vi "Two Color Servo Camera.vi"() -> ()   [LabVIEW 2013]
doc: "<B>Two Color Servo Camera </B> tracks a pink/green object by moving a gimbal mounted camera to keep the object centered in the image. It assumes the camera is mounted upright, and that the DS is connected. It is written to control two servos, but will work fine with one."
uses:
  <vilib>/addons/control/pid/pid.llb/PID Control Input Filter (DBL).vi
  <vilib>/Rock Robotics/WPI/Camera/WPI_CameraImageSize.ctl
  <vilib>/Rock Robotics/WPI/Camera/WPI_CameraWhite Balance Values.ctl
  <vilib>/Rock Robotics/WPI/Camera/WPI_CameraExposure Values.ctl
  Control Statesv1.ctl
  <vilib>/Rock Robotics/SystemInterfaces/DIO/FPGA_DIOPWMChannel.ctl
  <vilib>/Rock Robotics/WPI/Camera/WPI_CameraFrameRate.ctl
panel:
  in  "stop":bool
  in  "Frame Rate (fps)":T1=15 min=1 max=30
  out "Target":T2
  in  "Brightness":i32=40 min=0 max=100
  out "fps":dbl
  in  "Pink First":bool=TRUE
  in  "Friend Colors":enum32{"Pink over Green", "Green over Pink"}(radio)
  in  "Adv Processing Inputs":T3={"SubRect"={"Left"=0, "Top"=0, "Right"=640, "Bottom"=480}, "Decimate"={"H"=1, "V"=1}} {"Decimate"."V" min=1 max=1000; "Decimate"."H" min=1 max=1000}
  in  "Color Thresholds":T4(array[cluster])=[{"Hue"={"Min"=220, "Max"=255}, "Sat"={"Min"=75, "Max"=255}, "Luma"={"Min"=85, "Max"=255}}, {"Hue"={"Min"=55, "Max"=125}, "Sat"={"Min"=58, "Max"=255}, "Luma"={"Min"=92, "Max"=255}}]
  in  "Image Processing Limits":T5={"Find Foe"=TRUE, "Max Time (sec)"=0.25, "Min Obj Size %"=0.005, "Max Particles"=10}
  in  "Operation":enum32{"Camera Display", "Gimbal Track"}(radio)
  out "Servo Tracking State":T7
  in  "Servo Positions":cluster{"X":dbl, "Y":dbl}={"X"=85.52840986947938, "Y"=85.0} {"Y" scale=0.0..170.0; "X" scale=0.0..170.0}
  in  "Y Channel":T8=enum."PWM 10"
  in  "Servo Sleep (ms)":u32=20
  in  "X Channel":T8=enum."PWM 9"
  in  "Smooth":bool=TRUE
  out "Mask":T9(plugin-control)
  in  "Display Mask":bool=TRUE
  out "Camera Image":T9(plugin-control)
  # "This example will track a pink/green object by moving a gimbal mounted camera to keep the object centered in the image. It assumes the camera is mounted upright, and that the DS is connected. It is written to control two servos, but will work fine with one.\n\nThe setup code for the camera assumes that it is plugged into the switch and set to 10.te.am.11. To use on port 2 of an 8-slot controller, change the IP address wired into open.\n\nTo fine tune the colors, you may find it easiest to set the Operation control to Camera Display. This way the servos will not update and you can experiment with the colors or camera brightness  to get a good mask. Once the color thresholds are set appropriately for the object you are tracking, switch Operation to Gimbal Track."
  # "Servo Settings"
  # "Limit processing to a friend or foe,\nto a maximum amount of time,\nto particles above a minimum\nsize, and to a maximum number of color\nparticles"
  # "SubRect and decimate are used\nto limit the number of pixels to\nprocess. SubRect will for example\nextract the upper half of the\nimage. Decimate shrinks the image\nby for example leaving out every\nother row if V is set to 2."
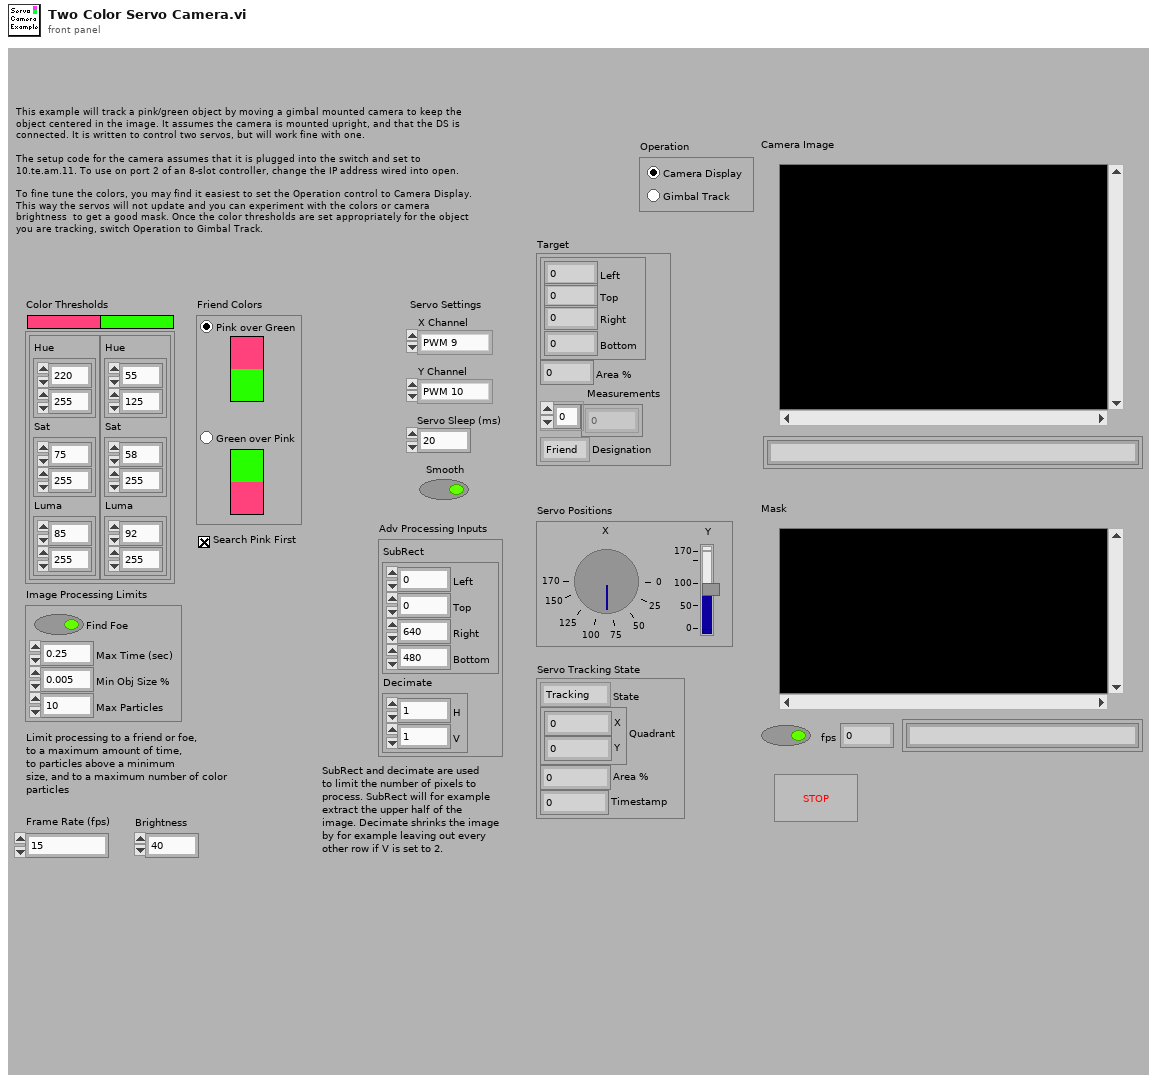
[diagram p1: front panel]
types:
  T1 = typedef "WPI_CameraFrameRate.ctl" = u32
  T2 = cluster{"Rectangle":cluster{"Left":i32, "Top":i32, "Right":i32, "Bottom":i32}, "Area %":dbl, "Measurements":dbl[], "Designation":enum16{"Friend", "Foe"}}
  T3 = cluster{"SubRect":cluster{"Left":i32, "Top":i32, "Right":i32, "Bottom":i32}, "Decimate":cluster{"H":i32, "V":i32}}
  T4 = cluster{"Hue":cluster{"Min":i32, "Max":i32}, "Sat":cluster{"Min":i32, "Max":i32}, "Luma":cluster{"Min":i32, "Max":i32}}[]
  T5 = cluster{"Find Foe":bool, "Max Time (sec)":dbl, "Min Obj Size %":sgl, "Max Particles":i32}
  T6 = typedef "Control Statesv1.ctl" = enum16{"Tracking", "Lost Small", "Lost-Patience", "Search-Begin", "Searching", "Lost - Edge"}
  T7 = cluster{"State":T6, "Quadrant":cluster{"X":i32, "Y":i32}, "Area %":dbl, "Timestamp":u32}
  T8 = typedef "FPGA_DIOPWMChannel.ctl" = enum8{"PWM 1", "PWM 2", "PWM 3", "PWM 4", "PWM 5", "PWM 6", "PWM 7", "PWM 8", "PWM 9", "PWM 10", "Invalid"}
  T9 = typedef "IMAQ Image.ctl" = refnum<image>
  T10 = typedef "WPI_CameraExposure Values.ctl" = enum16{"Auto", "Flicker-free 50 Hz", "Flicker-free 60 Hz", "Hold current"}
  T11 = typedef "WPI_CameraWhite Balance Values.ctl" = enum16{"Auto", "Fixed indoor", "Fixed outdoor 1", "Fixed outdoor 2", "Fixed fluorescent 1", "Fixed fluorescent 2", "Hold current"}
  T12 = typedef "WPI_CameraImageSize.ctl" = enum16{"640x480", "320x240", "160x120"}
  T13 = typedef "WPI_CameraDevRef.ctl" = cluster{"Camera Address":string, "CameraStatus":errorcluster, "Acquire Image Notifier":refnum<notifier>}
  T14 = cluster{"Image Processing Limits":cluster{"Find Foe":bool, "Max Time (sec)":dbl, "Min Obj Size %":sgl, "Max Particles":i32}, "Image Size":T12, "Pink First":bool}
  T15 = cluster{"State":T6, "Quadrant":cluster{"X":i32, "Y":i32}, "Area":dbl, "millisecond timer value":u32}
  T16 = typedef "WPI_ServoDeviceRef.ctl" = cluster{"DeviceStatus":errorcluster, "Digital Module":T17, "PWM Channel":T8, "DeadBand":T18}
  T17 = typedef "FPGA_TypedefDigitalModule.ctl" = enum16{"Digital Module 1", "Digital Module 2"}
  T18 = typedef "WPI_PWMDeadband.ctl" = cluster{"Name":string, "maxPositivePwm":i32, "minPositivePwm":i32, "centerPwm":i32, "maxNegativePwm":i32, "minNegativePwm":i32, "angularRange":u16}
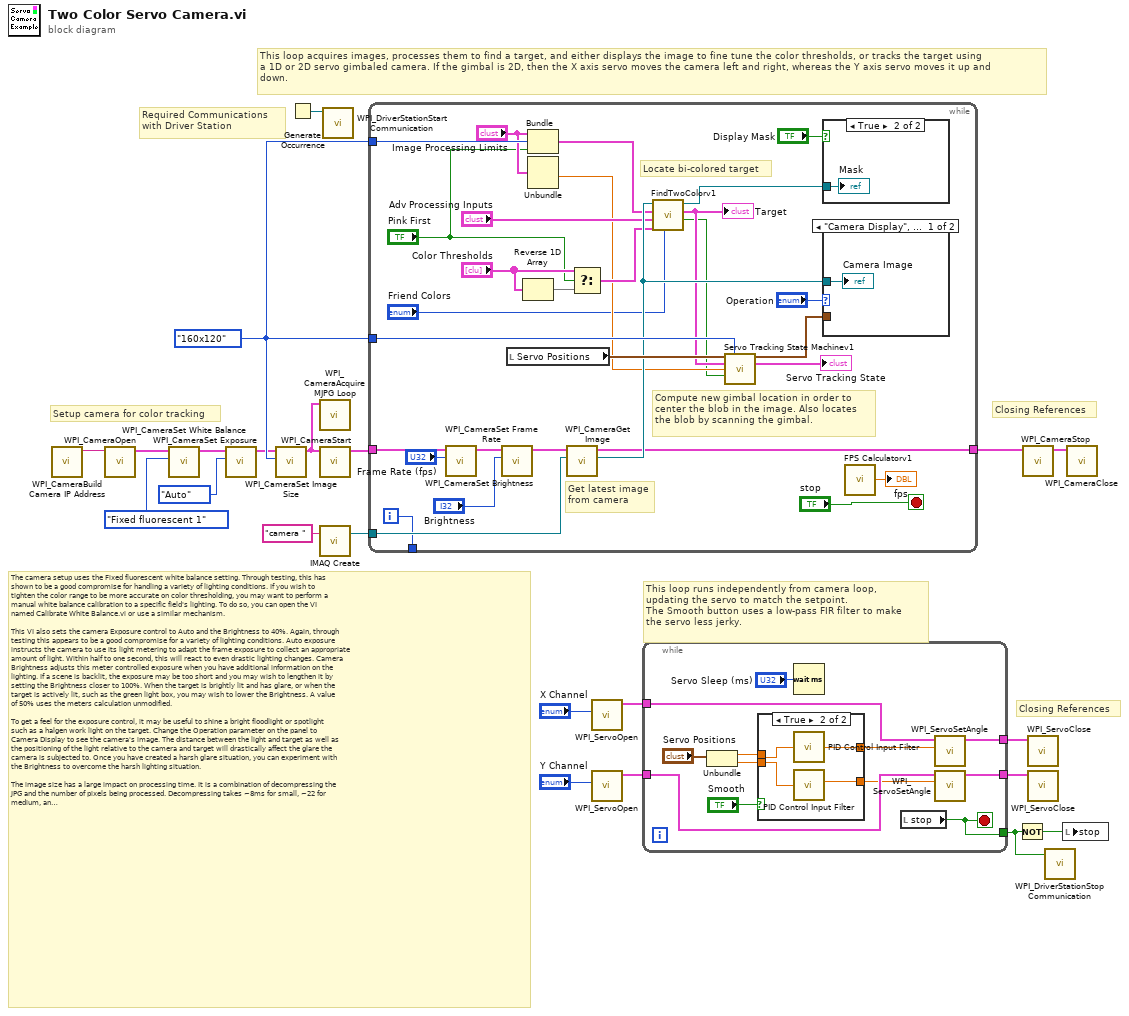
[diagram p0: block diagram]
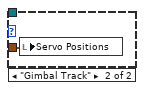
[diagram p3: hidden frame]
diagram:
  w13 = WPI_CameraImageSize."160x120" ("Image Size")
  # "Closing References"
  # "The camera setup uses the Fixed fluorescent white balance setting. Through testing, this has\nshown to be a good compromise for handling a variety of lighting conditions. If you wish to\ntighten the color range to be more accurate on color thresholding, you may want to perform a\nmanual white balance calibration to a specific field's lighting. To do so, you can open the VI\nnamed Calibrate White Balance.vi or use a similar mechanism.\n\nThis VI also sets the camera Exposure control to Auto and the Brightness to 40%. Again, through\ntesting this appears to be a good compromise for a variety of lighting conditions. Auto exposure\ninstructs the camera to use its light metering to adapt the frame exposure to collect an appropriate\namount of light. Within half to one second, this will react to even drastic lighting changes. Camera\nBrightness adjusts this meter controlled exposure when you have additional information on the\nlighting. If a scene is backlit, the exposure may be too short and you may wish to lengthen it by\nsetting the Brightness closer to 100%. When the target is brightly lit and has glare, or when the\ntarget is actively lit, such as the green light box, you may wish to lower the Brightness. A value\nof 50% uses the meters calculation unmodified.\n\nTo get a feel for the exposure control, it may be useful to shine a bright floodlight or spotlight\nsuch as a halgen work light on the target. Change the Operation parameter on the panel to\nCamera Display to see the camera's image. The distance between the light and target as well as\nthe positioning of the light relative to the camera and target will drastically affect the glare the\ncamera is subjected to. Once you have created a harsh glare situation, you can experiment with\nthe Brightness to overcome the harsh lighting situation.\n\nThe image size has a large impact on processing time. It is a combination of decompressing the\nJPG and the number of pixels being processed. Decompressing takes ~8ms for small, ~22 for\nmedium, and ~100 for large. After decompression, the processing time for locating targets is\nlargely related to the number of pixels. You may want to use the subRect or decimation factors\nto control the pixels being processed. Lower resolution or decimated images will be less effective\nat finding targets at distance."
  # "Closing References"
  # "This loop acquires images, processes them to find a target, and either displays the image to fine tune the color thresholds, or tracks the target using\na 1D or 2D servo gimbaled camera. If the gimbal is 2D, then the X axis servo moves the camera left and right, whereas the Y axis servo moves it up and\ndown."
  # "This loop runs independently from camera loop,\nupdating the servo to match the setpoint.\nThe Smooth button uses a low-pass FIR filter to make\nthe servo less jerky."
  # "Setup camera for color tracking"
  # "Required Communications\nwith Driver Station"
  n1 = call <vilib>:"WPI_CameraBuild Camera IP Address.vi"() -> ("Camera Address"=w3:string)  [unwired: 11 in]
  n2 = call <vilib>:"WPI_CameraOpen.vi"("Camera Address"=w3) -> ("CameraDevRef"=w11:T13)  [unwired: 1 in, 9 out]
  n3 = call <vilib>:"WPI_CameraSet White Balance.vi"("White Balance"=WPI_CameraWhite_Balance_Values."Fixed fluorescent 1", "CameraDevRef"=w11) -> ("CameraDevRef Out"=w9:T13)  [unwired: 1 in, 8 out]
  n4 = call <vilib>:"WPI_CameraSet Exposure.vi"("Exposure"=WPI_CameraExposure_Values."Auto", "CameraDevRef"=w9) -> ("CameraDevRef Out"=w4:T13)  [unwired: 1 in, 8 out]
  n5 = call <vilib>:"WPI_CameraSet Image Size.vi"("Image Size"=w13, "CameraDevRef"=w4) -> ("CameraDevRef Out"=w5:T13)  [unwired: 1 in, 8 out]
  n6 = Generate Occurrence() -> (w12:refnum<k4>)
  n7 = call <vilib>:"WPI_CameraAcquire MJPG Loop.vi"("CameraDevRef"=w5) -> ()  [unwired: 11 in]
  n8 = call <vilib>:"WPI_CameraStart.vi"("CameraDevRef"=w5) -> ("CameraDevRef Out"=w15:T13)  [unwired: 1 in, 9 out]
  n9 = call "IMAQ Create"("Image Name"="camera ") -> ("New Image"=w16:T9)  [unwired: 3 in, 2 out]
  n10 = call <vilib>:"WPI_DriverStationStart Communication.vi"("occurrence"=w12) -> ()  [unwired: 11 out]
  n11 = while {
    tunnel: w15 -> [w27]
    tunnel: [w36] -> w14
    tunnel: w16 -> [w52]
    tunnel: w13 -> [w48]
    tunnel: w13 -> [w39]
    tunnel: [w24] -> _
    i -> [w24]
    stop <- "stop" stop-if-true
    # "Locate bi-colored target"
    # "Compute new gimbal location in order to\ncenter the blob in the image. Also locates\nthe blob by scanning the gimbal."
    # "Get latest image\nfrom camera"
    n12 = call <vilib>:"WPI_CameraSet Frame Rate.vi"("Frame Rate (fps)"="Frame Rate (fps)", "CameraDevRef"=w27) -> ("CameraDevRef Out"=w26:T13)  [unwired: 1 in, 8 out]
    n13 = call <vilib>:"WPI_CameraSet Brightness.vi"("Brightness"="Brightness", "CameraDevRef"=w26) -> ("CameraDevRef Out"=w33:T13)  [unwired: 1 in, 8 out]
    n14 = local read "Servo Positions"() -> (w49:cluster{"X":dbl, "Y":dbl})
    n15 = Reverse 1D Array(array="Color Thresholds") -> (reversed array=w41:T4)
    n16 = Bundle("Image Processing Limits"="Image Processing Limits", "Image Size"=w39, "Pink First"="Pink First") -> (w40:T14)  [unwired: 1 out]
    n17 = Unbundle("Image Processing Limits") -> ("Min Obj Size %"=w37:sgl)  [unwired: 3 out]
    n18 = call <vilib>:"WPI_CameraGet Image.vi"("Image"=w52, "CameraDevRef"=w33) -> ("Image Out"=w46:T9, "CameraDevRef Out"=w36:T13)  [unwired: 1 in, 7 out]
    n19 = Select(t="Color Thresholds", s="Pink First", f=w41) -> (s? t:f=w42:T4)
    n20 = call "FindTwoColorv1.vi"("Friend Colors"="Friend Colors", "Color Ranges"=w42, "Adv Processing Data"="Adv Processing Inputs", "Processing Data"=w40, "Color Image In"=w46) -> ("Found"=w28:bool, "Target"=w29:T2, "Mask Image"=w45:T9)  [unwired: 2 out]
    "Target" <- w29
    n21 = call "Servo Tracking State Machinev1.vi"("Servo Positions In"=w49, "Image Size"=w48, "Target"=w29, "Area Limit"=w37, "Found"=w28) -> ("Servo Positions"=w51:cluster{"X":dbl, "Y":dbl}, "Tracking State Info"=→"Servo Tracking State":T15)  [unwired: 2 in, 7 out]
    n22 = case shown="True" "Display Mask" {
      tunnel: w45 -> [_ w53]
      frame False {
      }
      frame True {
        "Mask" <- w53
      }
    }
    n23 = case shown="\"Camera Display\", Default" "Operation" {
      tunnel: w51 -> [_ w55]
      tunnel: w46 -> [w54 _]
      frame "Camera Display", Default {
        "Camera Image" <- w54
      }
      frame "Gimbal Track" {
        n24 = local write "Servo Positions"(w55) -> ()
      }
    }
    n25 = call "FPS Calculatorv1.vi"() -> ("fps"=→"fps":dbl)  [unwired: 1 out]
  }
  n26 = call <vilib>:"WPI_ServoOpen.vi"("PWM Channel"="X Channel") -> ("ServoDeviceRef"=w20:T16)  [unwired: 3 in, 7 out]
  n27 = call <vilib>:"WPI_ServoOpen.vi"("PWM Channel"="Y Channel") -> ("ServoDeviceRef"=w19:T16)  [unwired: 3 in, 7 out]
  n28 = while {
    tunnel: w20 -> [w65]
    tunnel: [w67] -> w7
    tunnel: w19 -> [w64]
    tunnel: [w63] -> w6
    tunnel: [w56] -> w1
    stop <- w56 stop-if-true
    n29 = Unbundle("Servo Positions") -> ("X"=w61:dbl, "Y"=w59:dbl)
    n30 = case shown="True" "Smooth" {
      tunnel: w61 -> [w69 w73]
      tunnel: [w69 w72] -> w60
      tunnel: w59 -> [w68 w71]
      tunnel: [w68 w70] -> w58
      frame False {
      }
      frame True {
        n31 = call-poly <vilib>:"PID Control Input Filter.vi"("input"=w73) -> ("output"=w72:dbl)  [unwired: 1 in, 3 out]
        n32 = call-poly <vilib>:"PID Control Input Filter.vi"("input"=w71) -> ("output"=w70:dbl)  [unwired: 1 in, 3 out]
      }
    }
    n33 = Wait (ms)(milliseconds to wait="Servo Sleep (ms)") -> ()  [unwired: 1 out]
    n34 = local read "stop"() -> (w56:bool)
    n35 = call <vilib>:"WPI_ServoSetAngle.vi"("Angle"=w60, "ServoDeviceRef"=w65) -> ("ServoDeviceRef"=w67:T16)  [unwired: 1 in, 8 out]
    n36 = call <vilib>:"WPI_ServoSetAngle.vi"("Angle"=w58, "ServoDeviceRef"=w64) -> ("ServoDeviceRef"=w63:T16)  [unwired: 1 in, 8 out]
  }
  n37 = Not(x=w1) -> (.not. x?=w2:bool)
  n38 = call <vilib>:"WPI_CameraStop.vi"("CameraDevRef"=w14) -> ("CameraDevRef Out"=w18:T13)  [unwired: 1 in, 9 out]
  n39 = call <vilib>:"WPI_ServoClose.vi"("MotorControlDevRef"=w7) -> ()  [unwired: 1 in, 10 out]
  n40 = call <vilib>:"WPI_ServoClose.vi"("MotorControlDevRef"=w6) -> ()  [unwired: 1 in, 10 out]
  n41 = call <vilib>:"WPI_DriverStationStop Communication.vi"("StopCommunication"=w1) -> ()  [unwired: 1 in, 10 out]
  n42 = local write "stop"(w2) -> ()
  n43 = call <vilib>:"WPI_CameraClose.vi"("CameraDevRef"=w18) -> ()  [unwired: 1 in, 10 out]
